vi "GetEquipmentAssets.vi"(8 "error in (no error)":errorcluster, 11 "service":refnum<class "IcmMessageService.lvclass">) -> (0 "error out":errorcluster, 3 "AssetNodes":T1[](array[typedef]))   [LabVIEW 2017]
uses:
  <vilib>/addons/InsightCM/MessageBus/MessageService/IcmMessageService.lvclass
  <vilib>/addons/InsightCM/MessageBus/Base/controls/AssetNodeView.ctl
  <vilib>/addons/InsightCM/MessageBus/Base/controls/AssetState.ctl
  <vilib>/addons/InsightCM/MessageBus/Base/controls/Metric.ctl
  <vilib>/addons/InsightCM/MessageBus/Base/controls/KeyValuePair.ctl
  <vilib>/addons/InsightCM/MessageBus/Base/controls/AssetNodeReference.ctl
  <vilib>/addons/InsightCM/MessageBus/MessageLibrary/AssetManager/controls/AssetMgrQueryAssetNodeListRequestBody.ctl
  <vilib>/addons/InsightCM/MessageBus/Base/controls/AssetNodeListQueryParams.ctl
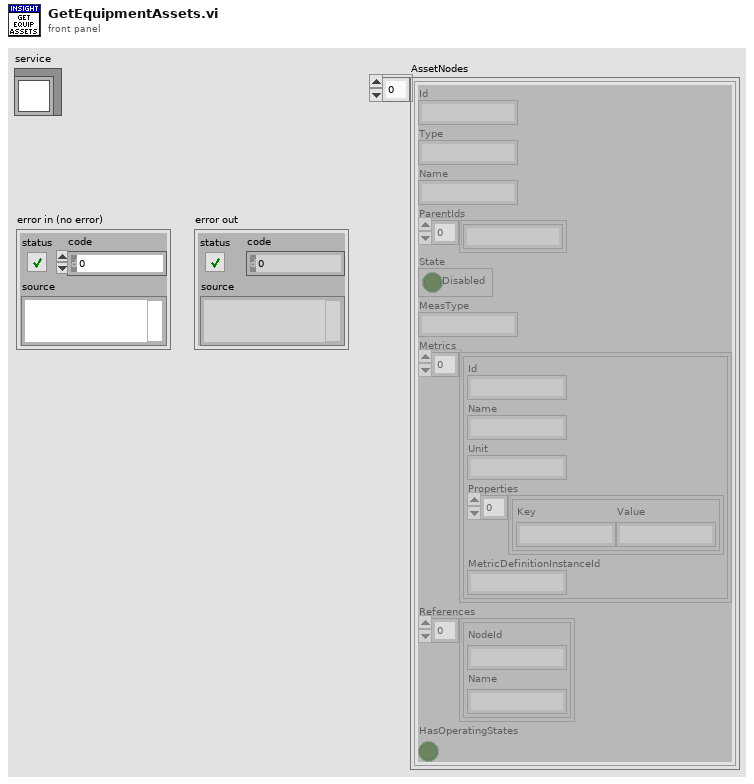
[diagram p1: front panel]
types:
  T1 = typedef "AssetNodeView.ctl" = cluster{"Id":string, "Type":string, "Name":string, "ParentIds":string[], "State":T2, "MeasType":string, "Metrics":T3[], "References":T5[], "HasOperatingStates":bool}
  T2 = typedef "AssetState.ctl" = cluster{"Disabled":bool}
  T3 = typedef "Metric.ctl" = cluster{"Id":string, "Name":string, "Unit":string, "Properties":T4[], "MetricDefinitionInstanceId":string}
  T4 = typedef "KeyValuePair.ctl" = cluster{"Key":string, "Value":string}
  T5 = typedef "AssetNodeReference.ctl" = cluster{"NodeId":string, "Name":string}
  T6 = typedef "AssetMgrQueryAssetNodeListRequestBody.ctl" = cluster{"QueryParams":T7}
  T7 = typedef "AssetNodeListQueryParams.ctl" = cluster{"Type":string, "MeasType":string, "Name":string, "Category":string, "PropKey":string, "PropValue":string, "HasOperatingStates":bool, "NeedsMapping":bool, "HasMetric":string, "Skip":i32, "Take":i32}
  T8 = typedef "Message.ctl" = cluster{"Header":T9, "Body":u8[]}
  T9 = typedef "MessageHeader.ctl" = cluster{"MessageName":string, "Timestamp":i64, "CorrelationId":string, "ContentType":string, "RoutingKey":string, "Properties":T4[]}
  T10 = typedef "AssetMgrQueryAssetNodeListResponseBody.ctl" = cluster{"AssetNodes":T1[], "TotalCount":i32}
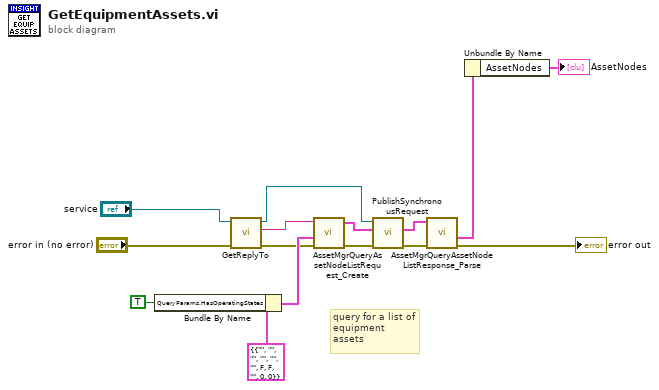
[diagram p0: block diagram]
diagram:
  # "query for a list of equipment assets"
  n1 = Bundle By Name(cluster=T6 {"QueryParams"={"Type"="", "MeasType"="", "Name"="", "Category"="", "PropKey"="", "PropValue"="", "HasOperatingStates"=FALSE, "NeedsMapping"=FALSE, "HasMetric"="", "Skip"=0, "Take"=0}} ("AssetMgrQueryAssetNodeListRequest"), "QueryParams.HasOperatingStates"=TRUE) -> (w13:T6)
  n2 = call <vilib>:"GetReplyTo.vi"("error in (no error)"="error in (no error)", "service in"="service") -> ("error out"=w10:errorcluster, "reply to"=w8:string, "service out"=w12:refnum<class "IcmMessageService.lvclass">)  [unwired: 7 in]
  n3 = call <vilib>:"AssetMgrQueryAssetNodeListRequest_Create.vi"("error in (no error)"=w10, "AssetMgrQueryAssetNodeListRequest"=w13, "ReplyTo"=w8) -> ("error out"=w11:errorcluster, "Message"=w9:T8)  [unwired: 7 in]
  n4 = call <vilib>:"PublishSynchronousRequest.vi"("error in (no error)"=w11, "request"=w9, "service in"=w12) -> ("error out"=w7:errorcluster, "response"=w5:T8)  [unwired: 6 in, 1 out]
  n5 = call <vilib>:"AssetMgrQueryAssetNodeListResponse_Parse.vi"("error in (no error)"=w7, "Message"=w5) -> ("error out"=→"error out":errorcluster, "Body"=w4:T10)  [unwired: 6 in, 2 out]
  n6 = Unbundle By Name(w4) -> ("AssetNodes"=→"AssetNodes":T1[])
